vi "testCalcUkInLsst.vi"(8 "error in (no error)":errorcluster) -> (0 "error out":errorcluster)   [LabVIEW 2016]
doc: "Test to calculate uk for LSST corner wavefront front sensor (WFS)."
uses:
  ZTAAC/ZTAAC.lvclass
  StrictDef/FilterType.ctl
  StrictDef/InstName.ctl
  <vilib>/Analysis/BLAS.llb/dasum - Absolute Values Sum (DBL).vi
  OfcFunc.lvlib
  <vilib>/addons/_JKI Toolkits/Caraya/classes/Test/Test.lvclass
  <vilib>/Analysis/NI_AALBLAS.lvlib
  <vilib>/addons/_JKI Toolkits/Caraya/classes/Assert/Assert.lvclass
  MatOper/MatOper.lvclass
panel:
  in  "ZTAAC.lvclass":refnum<class "ZTAAC.lvclass">
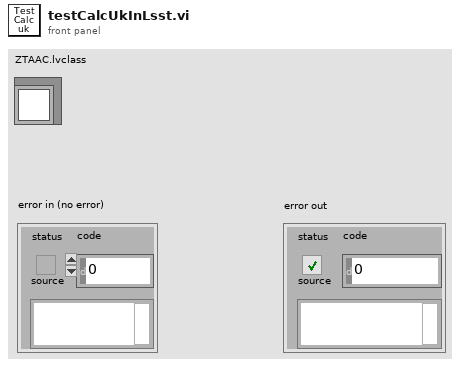
[diagram p1: front panel]
types:
  T1 = typedef "OfcFunc.lvlib/InstName.ctl" = enum16{"lsst", "comcam"}
  T2 = cluster{"Config Dir":path, "Inst Name":T1, "OptStateEsti Config File Name":string, "Mapping File Name":string, "Wavelength Table":string, "Intrinc Zk File Name":string, "y2 Corection File Name":string, "Index DOF File Name":string, "OptCtrl Config File Name":string, "State 0 File Name":string, "Weighting File Name":string, "PSSN Alpha File Name":string, "Authority Files":cluster{"Rigid Body Stroke File":string, "M1M3 Subsystem":cluster{"Mirror":string, "Actuatro Force File":string}, "M2 Subsystem":cluster{"Mirror":string, "Actuatro Force File":string}, "Num of Bending Mode":i32}, "Truncation Threshold":dbl}
  T3 = typedef "OfcFunc.lvlib/FilterType.ctl" = enum16{"ref", "u", "g", "r", "i", "z", "y"}
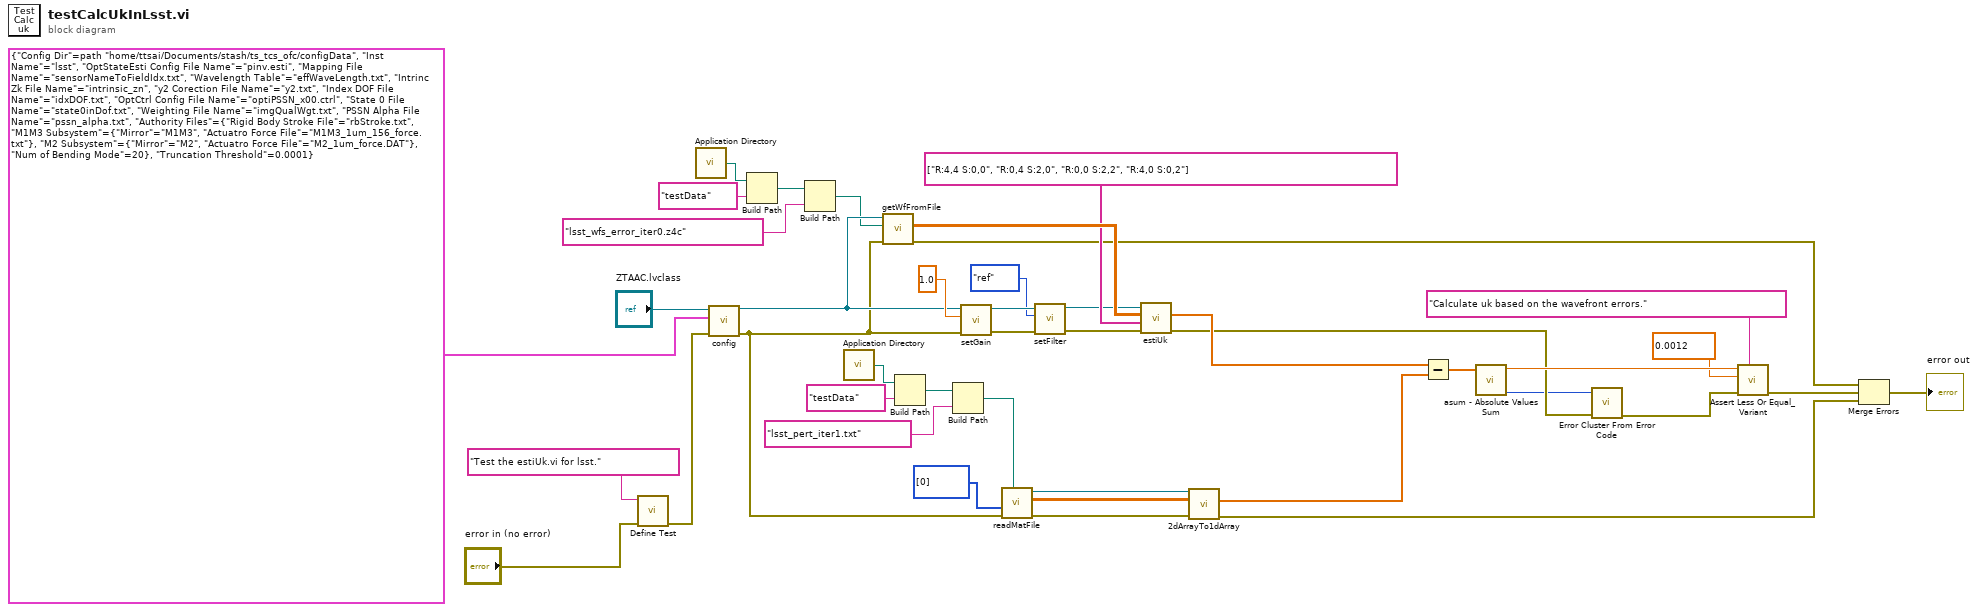
[diagram p0: block diagram]
diagram:
  n1 = call <vilib>:"Define Test.vi"("error in (no error)"="error in (no error)", "Label (VI Title)"="Test the estiUk.vi for lsst.") -> ("error out"=w35:errorcluster)  [unwired: 9 in]
  n2 = call <vilib>:"Application Directory.vi"() -> ("Application Directory"=w15:path)
  n3 = call "config.vi"("error in (no error)"=w35, "ZTAAC Configuration"=T2 {"Config Dir"=path "/home/ttsai/Documents/stash/ts_tcs_ofc/configData", "Inst Name"=enum."lsst", "OptStateEsti Config File Name"="pinv.esti", "Mapping File Name"="sensorNameToFieldIdx.txt", "Wavelength Table"="effWaveLength.txt", "Intrinc Zk File Name"="intrinsic_zn", "y2 Corection File Name"="y2.txt", "Index DOF File Name"="idxDOF.txt", "OptCtrl Config File Name"="optiPSSN_x00.ctrl", "State 0 File Name"="state0inDof.txt", "Weighting File Name"="imgQualWgt.txt", "PSSN Alpha File Name"="pssn_alpha.txt", "Authority Files"={"Rigid Body Stroke File"="rbStroke.txt", "M1M3 Subsystem"={"Mirror"="M1M3", "Actuatro Force File"="M1M3_1um_156_force.txt"}, "M2 Subsystem"={"Mirror"="M2", "Actuatro Force File"="M2_1um_force.DAT"}, "Num of Bending Mode"=20}, "Truncation Threshold"=0.0001}, "ZTAAC in"="ZTAAC.lvclass") -> ("error out"=w33:errorcluster, "ZTAAC out"=w40:refnum<class "ZTAAC.lvclass">)  [unwired: 7 in]
  n4 = Build Path(base path=w15, name or relative path="testData") -> (appended path=w13:path)
  n5 = Build Path(base path=w13, name or relative path="lsst_wfs_error_iter0.z4c") -> (appended path=w11:path)
  n6 = call <vilib>:"Application Directory.vi"() -> ("Application Directory"=w10:path)
  n7 = call "getWfFromFile.vi"("error in (no error)"=w33, "Wfs Err Data"=w11, "ZTAAC in"=w40) -> ("error out"=w32:errorcluster, "Wavefront Error"=w39:dbl[][])  [unwired: 6 in, 1 out]
  n8 = Build Path(base path=w10, name or relative path="testData") -> (appended path=w8:path)
  n9 = Build Path(base path=w8, name or relative path="lsst_pert_iter1.txt") -> (appended path=w6:path)
  n10 = call "setGain.vi"("error in (no error)"=w33, "Gain"=1.0, "ZTAAC in"=w40) -> ("error out"=w2:errorcluster, "ZTAAC out"=w5:refnum<class "ZTAAC.lvclass">)  [unwired: 7 in]
  n11 = call "readMatFile.vi"("Path"=w6, "error in (no error)"=w33, "Skip Col Idx"=i32[] [0] ("Skip Row Idx")) -> ("error out"=w17:errorcluster, "Matrix"=w37:dbl[][], "MatOper out"=w18:refnum<class "MatOper.lvclass">)  [unwired: 6 in]
  n12 = call "setFilter.vi"("error in (no error)"=w2, "Filter Type"=FilterType."ref", "ZTAAC in"=w5) -> ("error out"=w3:errorcluster, "ZTAAC out"=w4:refnum<class "ZTAAC.lvclass">)  [unwired: 7 in]
  n13 = call "estiUk.vi"("error in (no error)"=w3, "Sensor Name"=string[] ["R:4,4 S:0,0", "R:0,4 S:2,0", "R:0,0 S:2,2", "R:4,0 S:0,2"], "Wavefront Error"=w39, "ZTAAC in"=w4) -> ("error out"=w25:errorcluster, "uk Array"=w30:dbl[])  [unwired: 5 in, 1 out]
  n14 = call "2dArrayTo1dArray.vi"("error in (no error)"=w17, "2D Array"=w37, "MatOper in"=w18) -> ("error out"=w16:errorcluster, "1D Array"=w29:dbl[])  [unwired: 6 in, 1 out]
  n15 = Subtract(x=w30, y=w29) -> (x-y=w28:dbl[])
  n16 = call-poly <vilib>:"asum - Absolute Values Sum.vi"("x"=w28) -> ("error"=w24:i32, "dasum"=w27:dbl)  [unwired: 9 in]
  n17 = call <vilib>:"Error Cluster From Error Code.vi"("error in (no error)"=w25, "error code (0)"=w24) -> ("error out"=w23:errorcluster)  [unwired: 7 in]
  n18 = call <vilib>:"Assert Less Or Equal_Variant.vi"("Label"="Calculate uk based on the wavefront errors.", "error in (no error)"=w23, "Y"=0.0012, "X"=w27) -> ("error out"=w22:errorcluster)  [unwired: 7 in]
  n19 = Merge Errors(w32, w22, w16) -> (→"error out":errorcluster)
